vi "SingletonTemplate_GetObjectStatus.vi"(0 "reference in":refnum<class "SingletonTemplate.lvclass">, 5 "error in (no error)":errorcluster) -> (9 "Nr of users":i32, 10 "All objects names":string[](array[string]), 11 "One user":bool, 12 "# of objects":i32, 13 "Class name":string, 14 "reference out":refnum<class "SingletonTemplate.lvclass">, 15 "Not a refnum?":bool, 16 "Object name":string, 17 "All refs out":refnum<class "SingletonTemplate.lvclass">[](array[class]), 18 "Attributes locked?":bool, 19 "error out":errorcluster)   [LabVIEW 2012, in "SingletonTemplate.lvclass"]
doc: "Returns the object status and also information about all the objects in the class."
uses:
  <resource>/Framework/Providers/Open_GDS/ClassProviders/Provider_EndevoGOOP300/Templates/SingletonTemplate/SingletonTemplate.lvclass
  <vilib>/addons/_goop3.llb/3GOOPStates.ctl
  <resource>/Framework/Providers/Open_GDS/ClassProviders/Provider_EndevoGOOP300/Templates/SingletonTemplate/SingletonTemplate.lvclass/SingletonTemplate.ctl
panel:
  in  "DebuggerInput":string
  out "DebuggerOutput":string
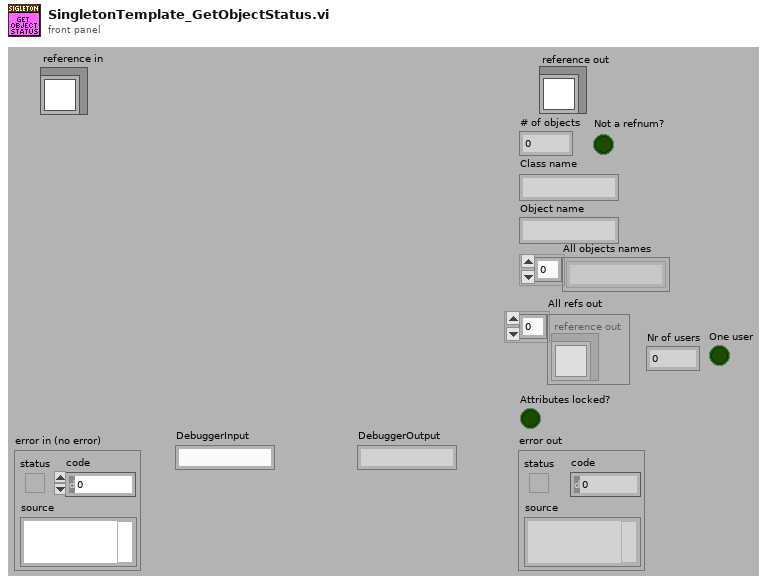
[diagram p1: front panel]
types:
  T1 = typedef "3GOOPStates.ctl" = enum16{"Set", "Get", "New", "Delete", "Clear", "Test and get", "Unlock data", "Information", "Look up existing", "New or look up existing", "Test and get shared", "Get shared", "Set shared", "Unlock shared", "Find dynamic method", "Register dynamic method", "Preload dynamic method", "Probe", "Cast to more generic", "Cast to more specific"}
  T2 = cluster{"Mode":enum16{"Get", "Set", "Delete"}, "Ref":i32, "ObjAttribute":string, "ClassAttribute":string}
  T3 = cluster{"Object names":string[], "Refs":i32[], "ObjectAttributeLocked":bool, "ClassAttributeLocked":bool, "ObjAttribute":variant, "ClassAttribute":variant}
  T4 = typedef "3GOOPClassStatistics.ctl" = cluster{"# of waiting":u32, "Object names":string[], "Base class folders":path[], "Refs":i32[], "Class name":string}
  T5 = typedef "SingletonTemplate.lvclass/ObjectAttributes.ctl" = cluster{"Attribute1":dbl}
  T6 = typedef "SingletonTemplate.lvclass/ClassAttributes.ctl" = cluster{"classAttribute1":bool}
  T7 = typedef "SingletonTemplate.lvclass/ObjectReference.ctl" = refnum<k1>
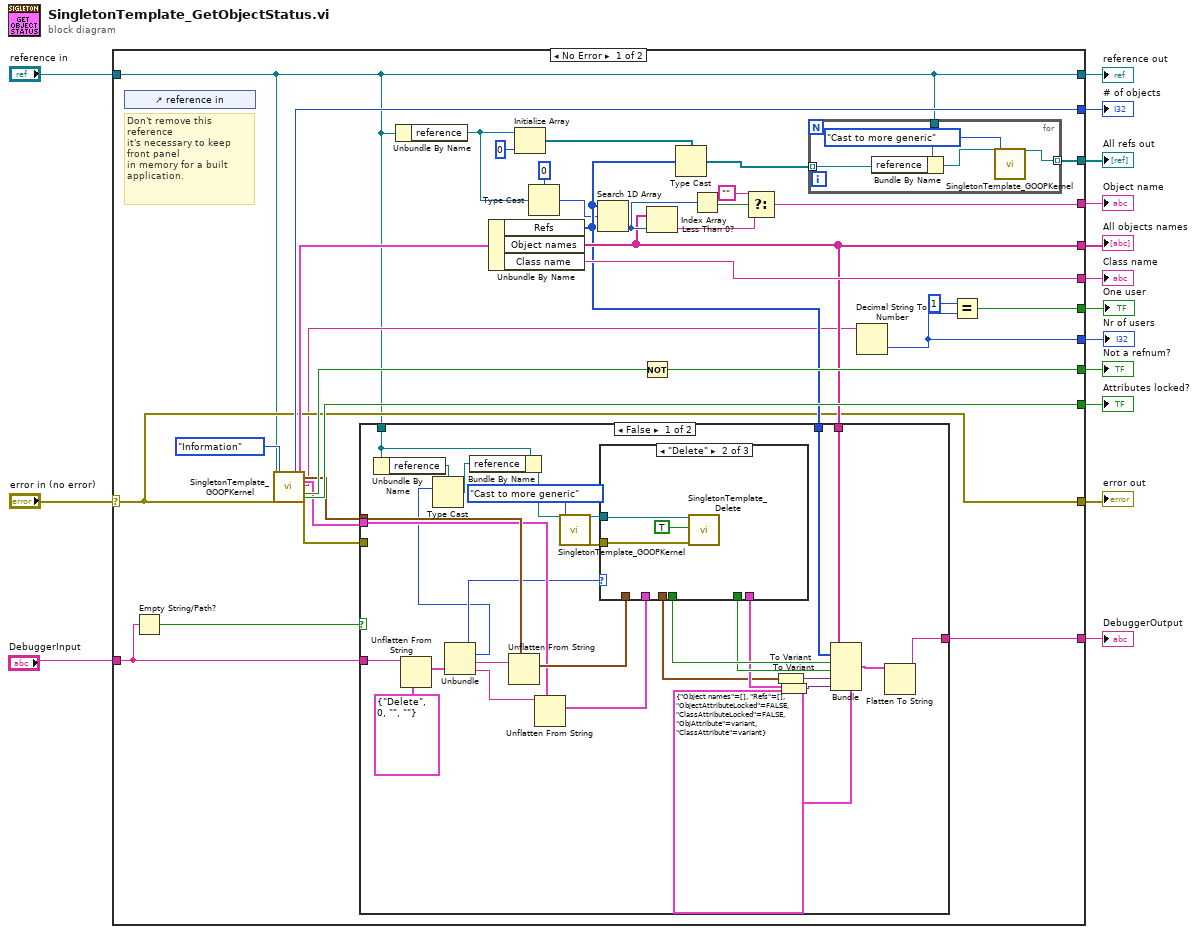
[diagram p0: block diagram]
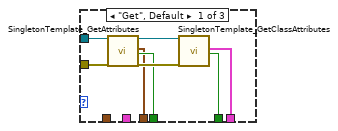
[diagram p2: hidden frame]
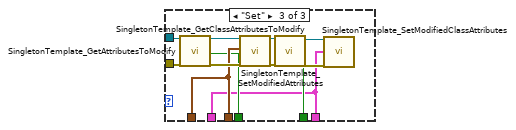
[diagram p3: hidden frame]
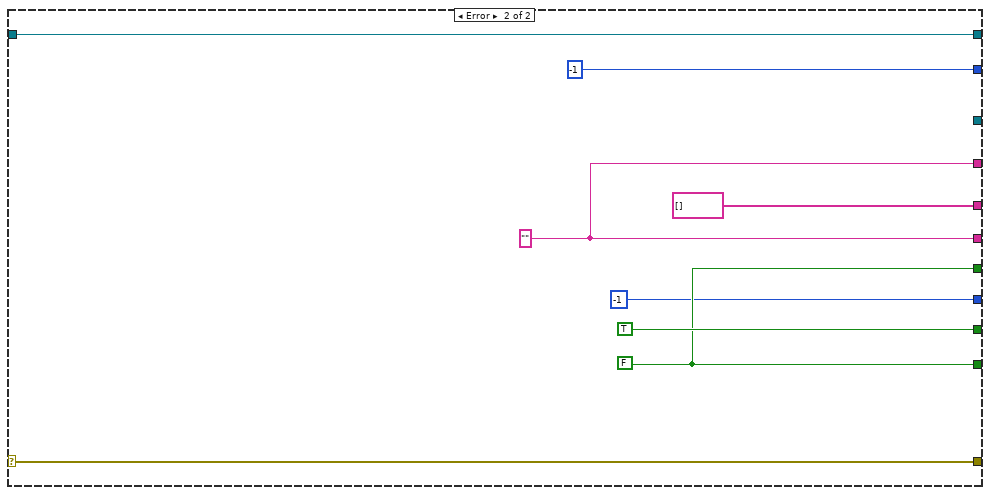
[diagram p5: hidden frame]
diagram:
  n1 = case shown="No Error" "error in (no error)" {
    selector: "error in (no error)" -> [w24 w113]
    tunnel: [w24 w113] -> w14
    tunnel: "reference in" -> [w16 w111]
    tunnel: [w16 w111] -> w12
    tunnel: [w47 -1 ("# of objects")] -> w11
    tunnel: [w43 TRUE ("Exists?")] -> w10
    tunnel: [w44 w107] -> w9
    tunnel: [w42 w108] -> w8
    tunnel: [w29 string[] [] ("Object names")] -> w7
    tunnel: [w25 _] -> w6
    tunnel: [w37 w108] -> w5
    tunnel: "DebuggerInput" -> [w34 _]
    tunnel: [w27 _] -> w3
    tunnel: [w22 -1] -> w2
    tunnel: [w21 w107] -> w1
    frame No Error {
      # "Don't remove this reference\nit's necessary to keep front panel\nin memory for a built application."
      n2 = control-ref of="reference in"() -> ()  [unwired: 1 out]
      n3 = Empty String/Path?(string/path=w34) -> (empty?=w33:bool)
      n4 = call <resource>:"SingletonTemplate_GOOPKernel.vi"("Ref in"=w16, "error in (no error)"=w24, "Action"=3GOOPStates."Information") -> ("# of objects"=w47:i32, "Class statistics"=w45:T4, "Data out"=w32:T5, "Data shared out"=w31:T6, "Probe out"=w23:string, "Exists?"=w46:bool, "Data locked?"=w44:bool, "error out"=w30:errorcluster)  [unwired: 14 in, 3 out]
      n5 = Unbundle By Name(w16) -> ("reference"=w17:T7)
      n6 = Unbundle By Name(w45) -> ("Refs"=w28:i32[], "Object names"=w29:string[], "Class name"=w42:string)
      n7 = case shown="False" w33 {
        tunnel: w30 -> [_ _]
        tunnel: w16 -> [w59 _]
        tunnel: [w78 _] -> w27
        tunnel: w32 -> [w73 _]
        tunnel: w31 -> [w72 _]
        tunnel: w34 -> [w70 _]
        tunnel: w28 -> [w68 _]
        tunnel: w29 -> [w67 _]
        frame False {
          n8 = Unbundle By Name(w59) -> ("reference"=w58:T7)
          n9 = Unflatten From String(type=T2 {"Mode"=enum."Delete", "Ref"=0, "ObjAttribute"="", "ClassAttribute"=""} ("DebuggerIn"), binary string=w70) -> (value=w75:T2)  [unwired: 3 in, 2 out]
          n10 = Unbundle(w75) -> ("Mode"=w71:enum16{"Get", "Set", "Delete"}, "Ref"=w60:i32, "ObjAttribute"=w76:string, "ClassAttribute"=w77:string)
          n11 = Type Cast(type=w58, x=w60) -> (*(type *) &x=w61:T7)
          n12 = Bundle By Name(cluster=w59, "reference"=w61) -> (w55:refnum<class "SingletonTemplate.lvclass">)
          n13 = Unflatten From String(type=w73, binary string=w76) -> (value=w74:T5)  [unwired: 3 in, 2 out]
          n14 = Unflatten From String(type=w72, binary string=w77) -> (value=w69:T6)  [unwired: 3 in, 2 out]
          n15 = call <resource>:"SingletonTemplate_GOOPKernel.vi"("Ref in"=w55, "Action"=3GOOPStates."Cast to more generic") -> ("Ref out"=w57:refnum<class "SingletonTemplate.lvclass">, "error out"=w56:errorcluster)  [unwired: 15 in, 9 out]
          n16 = case shown="\"Delete\"" w71 {
            tunnel: w56 -> [w90 w92 w104]
            tunnel: w57 -> [w89 w93 w105]
            tunnel: [w86 _ w96] -> w80
            tunnel: [w85 _ w95] -> w79
            tunnel: [w84 _ w97] -> w63
            tunnel: [w83 _ w94] -> w66
            tunnel: w74 -> [_ _ w97]
            tunnel: w69 -> [_ _ w94]
            frame "Get", Default {
              n17 = call <resource>:"SingletonTemplate_GetAttributes.vi"("reference in"=w89, "error in (no error)"=w90) -> ("reference out"=w88:refnum<class "SingletonTemplate.lvclass">, "Attributes"=w84:T5, "Attributes locked?"=w86:bool, "error out"=w87:errorcluster)  [unwired: 14 in]
              n18 = call <resource>:"SingletonTemplate_GetClassAttributes.vi"("reference in"=w88, "error in (no error)"=w87) -> ("Class attributes"=w83:T6, "Attributes locked?"=w85:bool)  [unwired: 14 in, 2 out]
            }
            frame "Delete" {
              n19 = call <resource>:"SingletonTemplate_Delete.vi"("reference in"=w93, "Force delete"=TRUE, "error in (no error)"=w92) -> ()  [unwired: 14 in, 3 out]
            }
            frame "Set" {
              n20 = call <resource>:"SingletonTemplate_GetAttributesToModify.vi"("reference in"=w105, "error in (no error)"=w104) -> ("reference out"=w103:refnum<class "SingletonTemplate.lvclass">, "Timeout"=w96:bool, "error out"=w102:errorcluster)  [unwired: 14 in, 1 out]
              n21 = call <resource>:"SingletonTemplate_SetModifiedAttributes.vi"("reference in"=w103, "Attributes"=w97, "error in (no error)"=w102) -> ("reference out"=w101:refnum<class "SingletonTemplate.lvclass">, "error out"=w100:errorcluster)  [unwired: 15 in]
              n22 = call <resource>:"SingletonTemplate_GetClassAttributesToModify.vi"("reference in"=w101, "error in (no error)"=w100) -> ("reference out"=w99:refnum<class "SingletonTemplate.lvclass">, "Timeout"=w95:bool, "error out"=w98:errorcluster)  [unwired: 14 in, 1 out]
              n23 = call <resource>:"SingletonTemplate_SetModifiedClassAttributes.vi"("reference in"=w99, "Class attributes"=w94, "error in (no error)"=w98) -> ()  [unwired: 15 in, 2 out]
            }
          }
          n24 = To Variant(anything=w63) -> (Variant=w64:variant)
          n25 = To Variant(anything=w66) -> (Variant=w65:variant)
          n26 = Bundle(cluster=T3 {"Object names"=[], "Refs"=[], "ObjectAttributeLocked"=FALSE, "ClassAttributeLocked"=FALSE, "ObjAttribute"=variant, "ClassAttribute"=variant}, "Object names"=w67, "Refs"=w68, "ObjectAttributeLocked"=w80, "ClassAttributeLocked"=w79, "ObjAttribute"=w64, "ClassAttribute"=w65) -> (w82:T3)
          n27 = Flatten To String(anything=w82) -> (data string=w78:string)  [unwired: 3 in, 2 out]
        }
        frame True {
        }
      }
      n28 = Initialize Array(w17, 0 ("Dimension Size")) -> (w35:T7[])
      n29 = Type Cast(type=0, x=w17) -> (*(type *) &x=w18:i32)
      n30 = Search 1D Array(1D array=w28, element=w18) -> (index of element=w41:i32)  [unwired: 1 in]
      n31 = Not(x=w46) -> (.not. x?=w43:bool)
      n32 = Index Array(array=w29, index=w41) -> (element=w39:string)
      n33 = Type Cast(type=w35, x=w28) -> (*(type *) &x=w26:T7[])
      n34 = Less Than 0?(x=w41) -> (x < 0?=w40:bool)
      n35 = Select(t="", s=w40, f=w39) -> (s? t:f=w37:string)
      n36 = for {
        tunnel: w26 -> [w53] mode=indexing
        tunnel: [w51] -> w25 mode=indexing
        tunnel: w16 -> [w49]
        n37 = Bundle By Name(cluster=w49, "reference"=w53) -> (w52:refnum<class "SingletonTemplate.lvclass">)
        n38 = call <resource>:"SingletonTemplate_GOOPKernel.vi"("Ref in"=w52, "Action"=3GOOPStates."Cast to more generic") -> ("Ref out"=w51:refnum<class "SingletonTemplate.lvclass">)  [unwired: 15 in, 10 out]
      }
      n39 = Decimal String To Number(string=w23) -> (number=w22:i32)  [unwired: 2 in, 1 out]
      n40 = Equal?(x=1, y=w22) -> (x = y?=w21:bool)
    }
    frame Error {
      w108 = "" ("Class name")
      w107 = FALSE
    }
  }
  "error out" <- w14
  "reference out" <- w12
  "# of objects" <- w11
  "Not a refnum?" <- w10
  "All refs out" <- w6
  "Attributes locked?" <- w9
  "Class name" <- w8
  "All objects names" <- w7
  "Object name" <- w5
  "DebuggerOutput" <- w3
  "One user" <- w1
  "Nr of users" <- w2
